vi "setup Write Out TGL LV.vi"(10 "outMsk":u16, 11 "instance":i32) -> ()   [LabVIEW 2022 SP3, in "SADI_FW3.lvlib"]
doc: "SADI_API_Wrapper void setupWrite_OutTGL_LV( int instance ,\n uint16_t outMsk );"
uses:
  SADI_FW3.lvlib
  SADI_FW3.dll
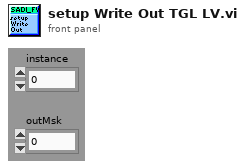
[diagram p1: front panel]
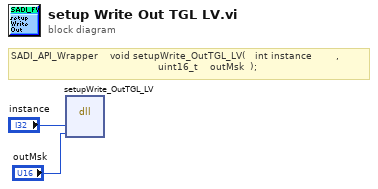
[diagram p0: block diagram]
diagram:
  # "SADI_API_Wrapper    void setupWrite_OutTGL_LV(   int instance        ,\n                                                 uint16_t    outMsk  );"
  n1 = dll-call lib="C:/Users/scer/OneDrive - University of Florida/eml4314c/eml4314SP23/resources/release_2_3_23/LV/LVLib/SADI_FW3.*" fn="setupWrite_OutTGL_LV"("instance"="instance", "outMsk"="outMsk") -> ()  [unwired: 6 in, 2 out]
